vi "Menu Selection.vi"(8 "error in (no error)":errorcluster, 10 "MenuTag":string, 11 "HIJ Vision Camera App In":refnum<class "HIJ Vision Camera App.lvclass">) -> (0 "error out":errorcluster, 3 "HIJ Vision Camera App Out":refnum<class "HIJ Vision Camera App.lvclass">)   [LabVIEW 2014, in "HIJ Vision Camera App.lvlib" / "HIJ Vision Camera App.lvclass"]
uses:
  HIJ Vision Camera App.lvclass
  HIJ Vision Camera App.lvclass/HIJ Vision Camera App.ctl
  HIJ Vision Camera App Dialog/HIJ Vision Camera App Dialog/HIJ Vision Camera App Dialog.lvclass/HIJ Vision Camera App Dialog.ctl
  HIJ Vision Camera App Dialog/HIJ Vision Camera App Dialog/Read Camera Name.vi
  HIJ Vision Camera App Dialog/HIJ Vision Camera App Dialog/HIJ Vision Camera App Dialog.lvclass
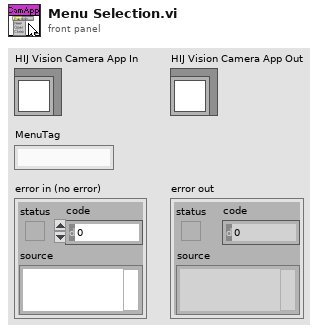
[diagram p1: front panel]
types:
  T1 = typedef "IMAQdx.ctl" = refnum<k21>
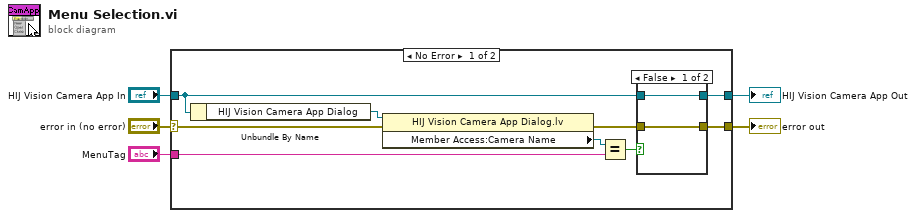
[diagram p0: block diagram]
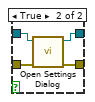
[diagram p2: hidden frame]
diagram:
  n1 = case shown="No Error" "error in (no error)" {
    selector: "error in (no error)" -> [w8 w22]
    tunnel: [w13 w22] -> w4
    tunnel: [w14 w21] -> w2
    tunnel: "HIJ Vision Camera App In" -> [w12 w21]
    tunnel: "MenuTag" -> [w10 _]
    frame No Error {
      n2 = Unbundle By Name(w12) -> ("HIJ Vision Camera App Dialog"=w11:refnum<class "HIJ Vision Camera App Dialog.lvclass">)
      n3 = property class="HIJ Vision Camera App Dialog.lv"(reference=w11, error in=w8) -> (error out=w7:errorcluster, "Member Access:Camera Name"=w9:T1)  [unwired: 1 out]
      n4 = Equal?(x=w9, y=w10) -> (x = y?=w6:bool)
      n5 = case shown="False" w6 {
        tunnel: [w16 w20] -> w14
        tunnel: [w15 w19] -> w13
        tunnel: w12 -> [w16 w18]
        tunnel: w7 -> [w15 w17]
        frame False {
        }
        frame True {
          n6 = call "Open Settings Dialog.vi"("error in (no error)"=w17, "HIJ Vision Camera App in"=w18) -> ("error out"=w19:errorcluster, "HIJ Vision Camera App out"=w20:refnum<class "HIJ Vision Camera App.lvclass">)  [unwired: 8 in]
        }
      }
    }
    frame Error {
    }
  }
  "error out" <- w4
  "HIJ Vision Camera App Out" <- w2
